vi "Recursively Get All Objects.vi"(8 "error in (no error)":errorcluster, 11 "AllObjs[] in":refnum<vi>[](array[refnum])) -> (0 "error out":errorcluster, 3 "AllObjs[] out":refnum<vi>[](array[refnum]))   [LabVIEW 2017, in "Open DQMH Request Message Diagram.lvlib"]
doc: "Recursively retrives all objects.\n\nBSD 3-Clause License\n\nCopyright (c) 2022, Neosoft Technologies Inc\nAll rights reserved.\n\nRedistribution and use in source and binary forms, with or without\nmodification, are permitted provided that the following conditions are met:\n\n1. Redistributions of source code must retain the above copyright notice, this\n list of conditions and the following disclaimer.\n\n2. Redistributions in binary form must reproduce the above copyright notice,\n this list of conditions and the following disclaimer in the documentation\n and/or other materials provided with the distribution.\n\n3. Neither the name of the copyright holder nor the names of its\n contributors may be used to endorse or promote products derived from\n this software without specific prior written permission.\n\nTHIS SOFTWARE IS PROVIDED BY THE COPYRIGHT HOLDERS AND CONTRIBUTORS \"AS IS\"\nAND ANY EXPRESS OR IMPLIED WARRANTIES, INCLUDING, BUT NOT LIMITED TO, THE\nIMPLIED WARRANTIES OF MERCHANTABILITY AND FITNESS FOR A PARTICULAR PURPOSE ARE\nDISCLAIMED. IN NO EVENT SHALL THE COPYRIGHT HOLDER OR CONTRIBUTORS BE LIABLE\nFOR ANY DIRECT, INDIRECT, INCIDENTAL, SPECIAL, EXEMPLARY, OR CONSEQUENTIAL\nDAMAGES (INCLUDING, BUT NOT LIMITED TO, PROCUREMENT OF SUBSTITUTE GOODS OR\nSERVICES; LOSS OF USE, DATA, OR PROFITS; OR BUSINESS INTERRUPTION) HOWEVER\nCAUSED AND ON ANY THEORY OF LIABILITY, WHETHER IN CONTRACT, STRICT LIABILITY,\nOR TORT (INCLUDING NEGLIGENCE OR OTHERWISE) ARISING IN ANY WAY OUT OF THE USE\nOF THIS SOFTWARE, EVEN IF ADVISED OF THE POSSIBILITY OF SUCH DAMAGE."
uses:
  Open DQMH Request Message Diagram.lvlib
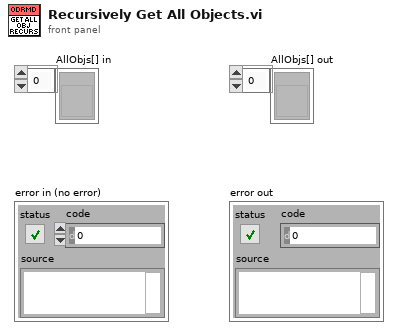
[diagram p1: front panel]
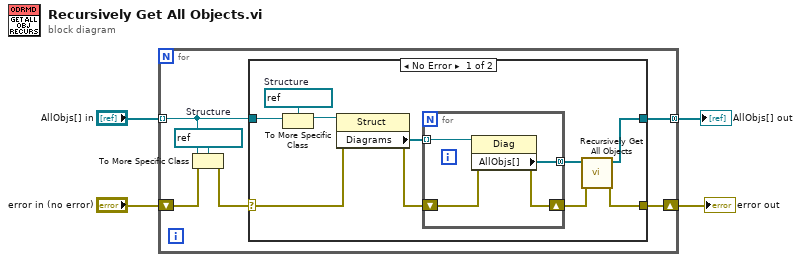
[diagram p0: block diagram]
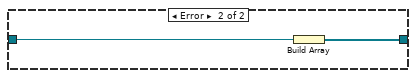
[diagram p2: hidden frame]
diagram:
  n1 = for {
    tunnel: "AllObjs[] in" -> [w6] mode=indexing
    tunnel: [w5] -> w1 mode=concatenating
    shift-right: [w7] -> w4
    shift-left: "error in (no error)" -> [w8]
    w10 = refnum<vi> refnum  # Structure
    n2 = To More Specific Class(target class=w10, reference=w6, error in=w8) -> (error out=w9:errorcluster)  [unwired: 1 out]
    n3 = case shown="No Error" w9 {
      selector: w9 -> [w20 _]
      tunnel: [w12 _] -> w7
      tunnel: w6 -> [w17 w26]
      tunnel: [w11 w25] -> w5
      frame No Error {
        w16 = refnum<vi> refnum  # Structure
        n4 = To More Specific Class(target class=w16, reference=w17) -> (specific class reference=w15:refnum<vi>)  [unwired: 1 in, 1 out]
        n5 = property class="Struct"(reference=w15, error in=w20) -> (error out=w18:errorcluster, "Diagrams"=w19:refnum<vi>[])  [unwired: 1 out]
        n6 = for {
          tunnel: w19 -> [w24] mode=indexing
          tunnel: [w23] -> w14 mode=concatenating
          shift-right: [w21] -> w13
          shift-left: w18 -> [w22]
          n7 = property class="Diag"(reference=w24, error in=w22) -> (error out=w21:errorcluster, "AllObjs[]"=w23:refnum<vi>[])  [unwired: 1 out]
        }
        n8 = call "Recursively Get All Objects.vi"("error in (no error)"=w13, "AllObjs[] in"=w14) -> ("error out"=w12:errorcluster, "AllObjs[] out"=w11:refnum<vi>[])  [unwired: 8 in]
      }
      frame Error {
        n9 = Build Array(w26) -> (w25:refnum<vi>[])
      }
    }
  }
  "error out" <- w4
  "AllObjs[] out" <- w1
